vi "init_RF_generators.vi"(5 "variables and parameter names":string[](array[string]), 7 "current variable and parameter values":dbl[](array[numeric]), 8 "error in":errorcluster, 11 "HP83623A Generator Settings Array":T1) -> (0 "error out":errorcluster)   [LabVIEW 2013, in "GPIB.lvclass"]
uses:
  GPIB.lvclass
  HP83623A_RF_Generator/HP83623A_array.ctl
  HP83623A_RF_Generator/HP83623A.ctl
  HP83623A_RF_Generator/HP83623A_RF_Generator.lvclass
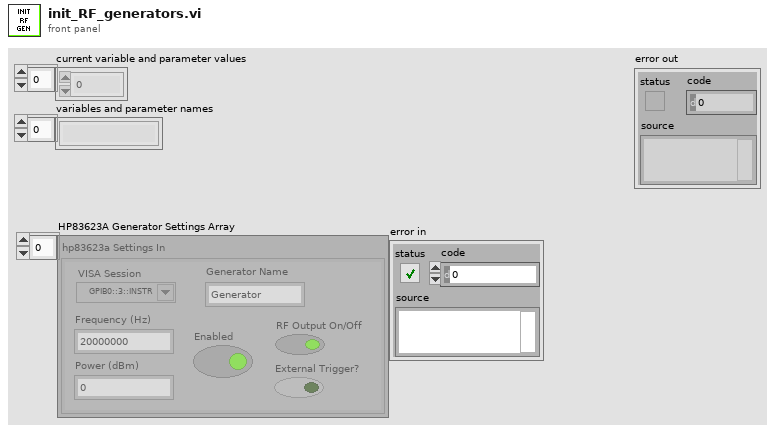
[diagram p1: front panel]
types:
  T1 = typedef "HP83623A_RF_Generator.lvclass/HP83623A_array.ctl" = T2[]
  T2 = typedef "HP83623A.ctl" = cluster{"Frequency (Hz)":string, "Power (dBm)":string, "Enabled":bool, "initialized":bool, "RF Output On/Off":bool, "External Trigger?":bool, "VISA Session":refnum<visa-resource-name>, "Generator Name":string}
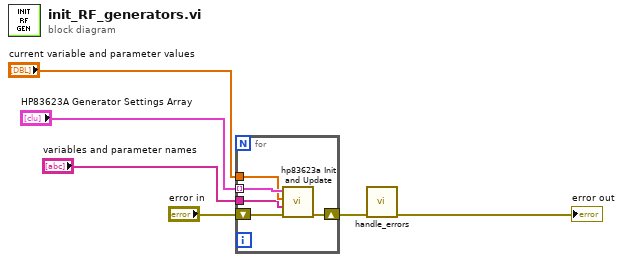
[diagram p0: block diagram]
diagram:
  n1 = for {
    shift-right: [w10] -> w2
    shift-left: "error in" -> [w11]
    tunnel: "HP83623A Generator Settings Array" -> [w9] mode=indexing
    tunnel: "current variable and parameter values" -> [w8]
    tunnel: "variables and parameter names" -> [w7]
    n2 = call "hp83623a Init and Update.vi"("error in (no error)"=w11, "Variable Names"=w7, "Variable Values"=w8, "hp83623a Settings In"=w9) -> ("error out"=w10:errorcluster)  [unwired: 6 in, 1 out]
  }
  n3 = call "handle_errors.vi"("error in (no error)"=w2) -> ("error out"=→"error out":errorcluster)  [unwired: 10 in]
